vi "FGV Gaszuordnung Grenzen&Einheiten.vi"(6 "Aktion":T1, 9 "Max":dbl[](array[numeric]), 10 "Min":dbl[](array[numeric])) -> (0 "Einheit neu":string[](array[string]), 1 "Max neu":dbl[](array[numeric]), 2 "Min neu":dbl[](array[numeric]), 3 "Namen neu":string[](array[string]))   [LabVIEW 2020, in "Gaszuordnung AO.lvlib"]
uses:
  Gaszuordnung AO.lvlib
  FGV Gaszuordnung Grenzen&Einheit Aktion.ctl
  Allgemein/allgemeine Sub-VIs.lvlib
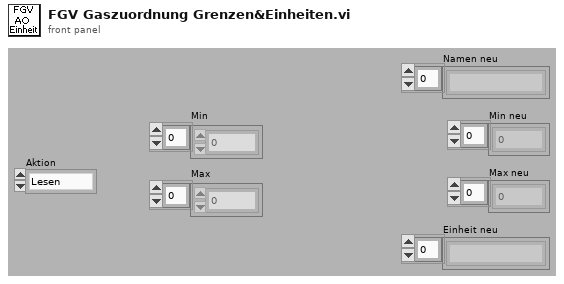
[diagram p1: front panel]
types:
  T1 = typedef "Gaszuordnung AO.lvlib/FGV Gaszuordnung Grenzen&Einheit Aktion.ctl" = enum16{"Lesen", "Schreiben Min", "Schreiben Max", "Laden", "Speichern"}
  T2 = enum16{"open", "replace", "create", "open or create", "replace or create", "replace or create with confirmation"}
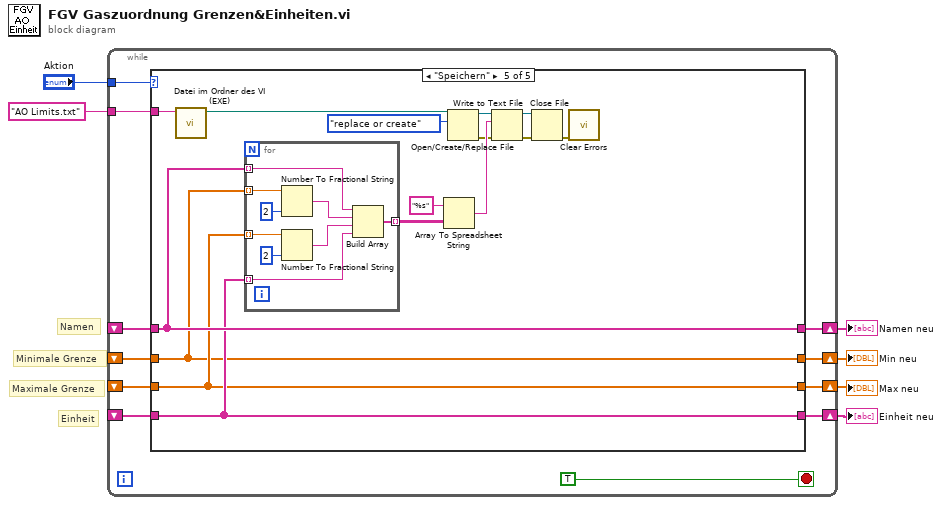
[diagram p0: block diagram]
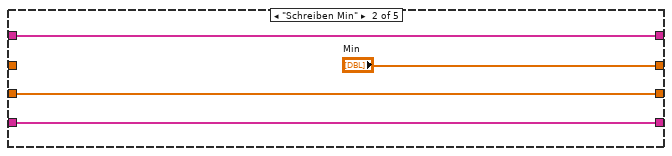
[diagram p3: hidden frame]
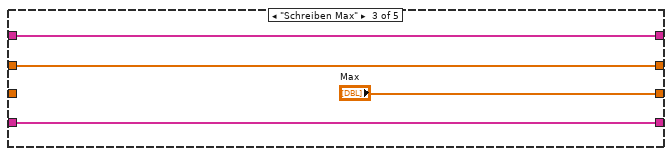
[diagram p4: hidden frame]
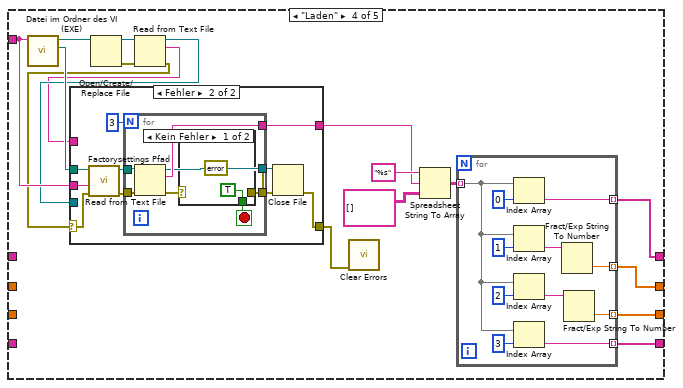
[diagram p5: hidden frame]
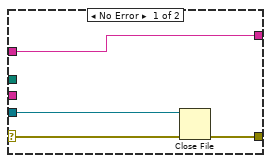
[diagram p6: hidden frame]
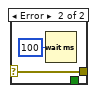
[diagram p7: hidden frame]
diagram:
  # "Einheit"
  # "Maximale Grenze"
  # "Minimale Grenze"
  # "Namen"
  n1 = while {
    shift-right: [w15] -> w4
    shift-left: _ -> [w11]
    tunnel: "Aktion" -> [w16]
    shift-right: [w14] -> w3
    shift-left: _ -> [w10]
    shift-right: [w13] -> w2
    shift-left: _ -> [w9]
    shift-right: [w12] -> w1
    shift-left: _ -> [w8]
    tunnel: "AO Limits.txt" ("Dateiname") -> [w7]
    stop <- TRUE stop-if-true
    n2 = case shown="\"Speichern\"" w16 {
      tunnel: [w21 w24 w28 w40 w87] -> w15
      tunnel: [w20 "Min" w27 w39 w84] -> w14
      tunnel: [w19 w23 "Max" w38 w85] -> w13
      tunnel: [w18 w22 w26 w37 w86] -> w12
      tunnel: w11 -> [w21 w24 w28 _ w87]
      tunnel: w10 -> [w20 _ w27 _ w84]
      tunnel: w9 -> [w19 w23 _ _ w85]
      tunnel: w8 -> [w18 w22 w26 _ w86]
      tunnel: w7 -> [_ _ _ w35 w95]
      frame "Lesen", Default {
      }
      frame "Schreiben Min" {
      }
      frame "Schreiben Max" {
      }
      frame "Laden" {
        n3 = call "Datei im Ordner des VI (EXE).vi"("Dateiname"=w35) -> ("Ordner des Haupt-VIs"=w36:path, "Dateipfad im Ordner des Haupt-VIs"=w46:path)  [unwired: 8 in, 1 out]
        n4 = Open/Create/Replace File(file path (use dialog)=w46) -> (refnum out=w44:refnum<file>, error out=w45:errorcluster)  [unwired: 1 in, 5 out]
        n5 = Read from Text File(file (use dialog)=w44, error in=w45) -> (refnum out=w34:refnum<file>, text=w33:string, error out=w30:errorcluster)  [unwired: 3 out]
        n6 = case shown="Fehler" w30 {
          selector: w30 -> [w49 w52]
          tunnel: w36 -> [_ w53]
          tunnel: w33 -> [w50 _]
          tunnel: [w50 w59] -> w32
          tunnel: [w47 w57] -> w31
          tunnel: w34 -> [w48 _]
          tunnel: w35 -> [_ w51]
          frame No Error {
            n7 = Close File(refnum=w48, error in=w49) -> (error out=w47:errorcluster)  [unwired: 1 out]
          }
          frame Error {
            n8 = call "Factorysettings Pfad.vi"("error in (no error)"=w52, "Dateiname"=w51, "Ordner des Haupt-VIs"=w53) -> ("error out"=w54:errorcluster, "Pfad Factorysettings"=w55:path)  [unwired: 7 in]
            n9 = for {
              N: 3 -> [_]
              tunnel: w54 -> [w65]
              tunnel: w55 -> [w64]
              tunnel: [w63] -> w59
              tunnel: [w62] -> w58
              tunnel: [w61] -> w56
              stop <- w66 stop-if-true
              n10 = Read from Text File(file (use dialog)=w64, error in=w65) -> (refnum out=w61:refnum<file>, text=w63:string, error out=w67:errorcluster)  [unwired: 2 in, 1 out]
              n11 = case shown="Kein Fehler" w67 {
                selector: w67 -> [_ w70]
                tunnel: [TRUE _] -> w66
                tunnel: [errorcluster {"status"=FALSE, "code"=0, "source"=""} ("error IO") w70] -> w62
                frame No Error {
                }
                frame Error {
                  n12 = Wait (ms)(milliseconds to wait=u32 100 ("Zu wartende ms")) -> ()  [unwired: 1 out]
                }
              }
            }
            n13 = Close File(refnum=w56, error in=w58) -> (error out=w57:errorcluster)  [unwired: 1 out]
          }
        }
        n14 = call <vilib>:"Clear Errors.vi"("error in (no error)"=w31) -> ()  [unwired: 5 in, 2 out]
        n15 = Spreadsheet String To Array(format string="%s" ("Format-String"), spreadsheet string=w32, array type (2D Dbl)=string[][] []) -> (array=w41:string[][])  [unwired: 1 out]
        n16 = for {
          tunnel: w41 -> [w82] mode=indexing
          tunnel: [w77] -> w40 mode=indexing
          tunnel: [w75] -> w39 mode=indexing
          tunnel: [w73] -> w38 mode=indexing
          tunnel: [w72] -> w37 mode=indexing
          n17 = Index Array(array=w82, index=0 ("Index")) -> (element=w77:string)
          n18 = Index Array(array=w82, index=1 ("Index")) -> (element=w76:string)
          n19 = Index Array(array=w82, index=2 ("Index")) -> (element=w74:string)
          n20 = Index Array(array=w82, index=3 ("Index")) -> (element=w72:string)
          n21 = Fract/Exp String To Number(string=w76) -> (number=w75:dbl)  [unwired: 4 out]
          n22 = Fract/Exp String To Number(string=w74) -> (number=w73:dbl)  [unwired: 4 out]
        }
      }
      frame "Speichern" {
        n23 = call "Datei im Ordner des VI (EXE).vi"("Dateiname"=w95) -> ("Dateipfad im Ordner des Haupt-VIs"=w94:path)  [unwired: 8 in, 2 out]
        n24 = for {
          tunnel: w87 -> [w102] mode=indexing
          tunnel: w84 -> [w106] mode=indexing
          tunnel: w85 -> [w103] mode=indexing
          tunnel: w86 -> [w99] mode=indexing
          tunnel: [w98] -> w97 mode=indexing
          n25 = Number To Fractional String(number=w106, precision (6)=i16 2 ("Genauigkeit (6)")) -> (F-format string=w101:string)  [unwired: 2 out]
          n26 = Number To Fractional String(number=w103, precision (6)=i16 2 ("Genauigkeit (6)")) -> (F-format string=w100:string)  [unwired: 2 out]
          n27 = Build Array(w102, w101, w100, w99) -> (w98:string[])
        }
        n28 = Array To Spreadsheet String(array=w97, 3:"%s" ("Format-String")) -> (spreadsheet string=w92:string)  [unwired: 1 out]
        n29 = Open/Create/Replace File(file path (use dialog)=w94, operation (0:open)=T2."replace or create" ("Operation (0:Öffnen)")) -> (refnum out=w93:refnum<file>, error out=w89:errorcluster)  [unwired: 1 in, 4 out]
        n30 = Write to Text File(file (use dialog)=w93, text=w92, error in=w89) -> (refnum out=w90:refnum<file>, error out=w91:errorcluster)  [unwired: 2 out]
        n31 = Close File(refnum=w90, error in=w91) -> (error out=w83:errorcluster)  [unwired: 1 out]
        n32 = call <vilib>:"Clear Errors.vi"("error in (no error)"=w83) -> ()  [unwired: 5 in, 2 out]
      }
    }
  }
  "Namen neu" <- w4
  "Min neu" <- w3
  "Max neu" <- w2
  "Einheit neu" <- w1
